vi "Ramp Up Voltage.vi"(8 "error in":errorcluster, 9 "V Ch 1":refnum<vi>, 10 "V Ch 0":refnum<vi>, 11 "BoardHandle in":T1) -> (0 "error out":errorcluster, 2 "BoardHandle out":T1)   [LabVIEW 2020]
uses:
  <instrlib>/CAEN PSM/CAEN PSM.lvlib
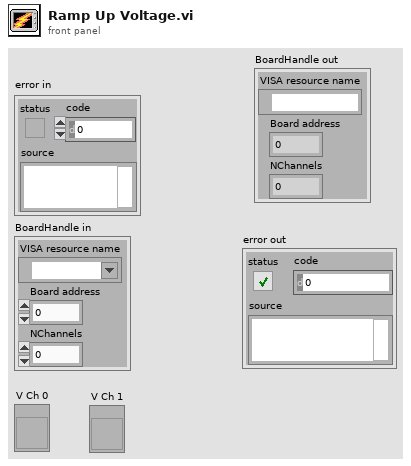
[diagram p1: front panel]
types:
  T1 = cluster{"VISA resource name":refnum<visa-resource-name>, "Board address":u8, "NChannels":u8}
  T2 = typedef "CAEN PSM.lvlib/BoardHandle.ctl" = cluster{"VISA resource name":refnum<visa-resource-name>, "Board address":i8, "NChannels":u8}
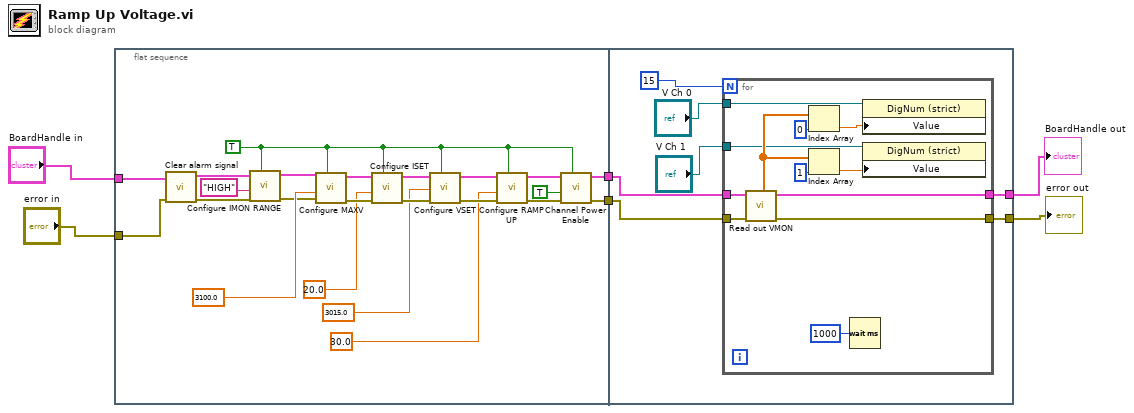
[diagram p0: block diagram]
diagram:
  n1 = flat-sequence {
    tunnel: [w17] -> w6
    tunnel: [w16] -> w5
    tunnel: "BoardHandle in" -> [w8]
    tunnel: "error in" -> [w7]
    tunnel: w6 -> [w35]
    tunnel: w5 -> [w34]
    tunnel: [w31] -> w2
    tunnel: [w30] -> w1
    frame #0 {
      w9 = TRUE ("All Channels (F)")
      n2 = call <instrlib>:"Clear alarm signal.vi"("error in (no error)"=w7, "BoardHandle"=w8) -> ("error out"=w14:errorcluster, "BoardHandle out"=w13:T2)  [unwired: 8 in]
      n3 = call <instrlib>:"Configure IMON RANGE.vi"("All Channels (F)"=w9, "error in (no error)"=w14, "IMon range (LOW)"="HIGH", "BoardHandle"=w13) -> ("error out"=w10:errorcluster, "BoardHandle out"=w11:T2)  [unwired: 6 in]
      n4 = call <instrlib>:"Configure MAXV.vi"("All Channels (F)"=w9, "error in (no error)"=w10, "Voltage Max (0.0 V)"=3100.0 ("VMax (Volts)"), "BoardHandle"=w11) -> ("error out"=w26:errorcluster, "BoardHandle out"=w23:T2)  [unwired: 6 in]
      n5 = call <instrlib>:"Configure ISET.vi"("All Channels (F)"=w9, "error in (no error)"=w26, "Current Limit (0.00 uA)"=20.0 ("Current Limit (uA)"), "BoardHandle"=w23) -> ("error out"=w27:errorcluster, "BoardHandle out"=w22:T2)  [unwired: 6 in]
      n6 = call <instrlib>:"Configure VSET.vi"("All Channels (F)"=w9, "error in (no error)"=w27, "Voltage Level (0.0 V)"=3015.0 ("Voltage Set (Volts)"), "BoardHandle"=w22) -> ("error out"=w28:errorcluster, "BoardHandle out"=w21:T2)  [unwired: 6 in]
      n7 = call <instrlib>:"Configure RAMP UP.vi"("All Channels (F)"=w9, "error in (no error)"=w28, "Voltage ramp up (0 V/s)"=30.0 ("Voltage Ramp Up (V/s)"), "BoardHandle"=w21) -> ("error out"=w29:errorcluster, "BoardHandle out"=w20:T2)  [unwired: 6 in]
      n8 = call <instrlib>:"Channel Power Enable.vi"("All Channels (F)"=w9, "error in (no error)"=w29, "Enable (OFF)"=TRUE ("Boolean"), "BoardHandle"=w20) -> ("error out"=w16:errorcluster, "BoardHandle out"=w17:T2)  [unwired: 6 in]
    }
    frame #1 {
      n9 = for {
        N: 15 -> [_]
        tunnel: w35 -> [w42]
        tunnel: w34 -> [w41]
        tunnel: "V Ch 0" -> [w40]
        tunnel: "V Ch 1" -> [w39]
        tunnel: [w38] -> w31
        tunnel: [w37] -> w30
        n10 = call <instrlib>:"Read out VMON.vi"("error in (no error)"=w41, "BoardHandle"=w42) -> ("error out"=w37:errorcluster, "VMon values (V)"=w43:dbl[], "BoardHandle out"=w38:T2)  [unwired: 7 in]
        n11 = Index Array(array=w43, index=0) -> (element=w46:dbl)
        n12 = Index Array(array=w43, index=1) -> (element=w44:dbl)
        n13 = Wait (ms)(milliseconds to wait=u32 1000) -> ()  [unwired: 1 out]
        n14 = property class="DigNum (strict)"(reference=w40, "Value"=w46) -> ()  [unwired: 1 in, 2 out]
        n15 = property class="DigNum (strict)"(reference=w39, "Value"=w44) -> ()  [unwired: 1 in, 2 out]
      }
    }
  }
  "BoardHandle out" <- w2
  "error out" <- w1
